vi "append filename to Cascade csv data file.vi"(10 "new ending (none)":string, 11 "Output File Path":path) -> (3 "Path":path)   [LabVIEW 2016]
uses:
  <userlib>/_OpenG.lib/file/file.llb/File Exists - Scalar__ogtk.vi
  <userlib>/_OpenG.lib/file/file.llb/Strip Path - Traditional__ogtk.vi
panel:
  out "Output File Path is directory 2":bool
  out "is directory":bool
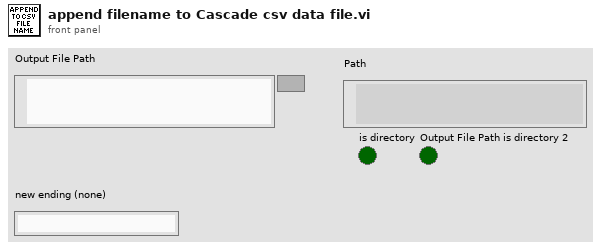
[diagram p1: front panel]
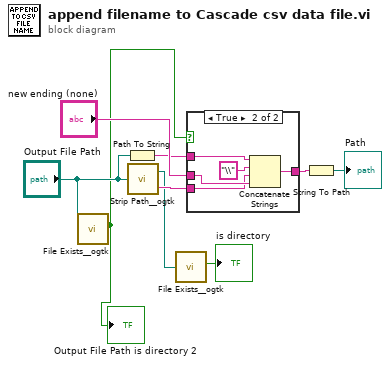
[diagram p0: block diagram]
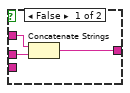
[diagram p2: hidden frame]
diagram:
  n1 = call-poly <userlib>:"File Exists__ogtk.vi"("file path"="Output File Path") -> ("is directory"=w1:bool)  [unwired: 6 in, 1 out]
  "Output File Path is directory 2" <- w1
  n2 = Path To String(path="Output File Path") -> (string=w6:string)
  n3 = call-poly <userlib>:"Strip Path__ogtk.vi"("path"="Output File Path") -> ("stripped path"=w3:path, "name"=w5:string)
  n4 = call-poly <userlib>:"File Exists__ogtk.vi"("file path"=w3) -> ("is directory"=→"is directory":bool)  [unwired: 6 in, 1 out]
  n5 = case shown="True" w1 {
    tunnel: "new ending (none)" -> [w12 w15]
    tunnel: [w11 w16] -> w7
    tunnel: w6 -> [w10 w17]
    tunnel: w5 -> [_ w14]
    frame False {
      n6 = Concatenate Strings(w10, w12) -> (w11:string)
    }
    frame True {
      n7 = Concatenate Strings(w17, "\\" ("string"), w14, w15) -> (w16:string)
    }
  }
  n8 = String To Path(string=w7) -> (path=→"Path":path)
